vi "Lower_Stop_ms2.vi"(8 "error in (no error)":errorcluster, 10 "I-O in":refnum<class "I-O.lvclass">, 11 "Motion in":refnum<class "Motion.lvclass">) -> (0 "error out":errorcluster, 2 "I-O out":refnum<class "I-O.lvclass">, 3 "Motion out":refnum<class "Motion.lvclass">)   [LabVIEW 2016]
uses:
  Classes/Controller/Motion/Motion Folder/Motion.lvclass
  Classes/Controller/I-O/I-O Folder/I-O.lvclass
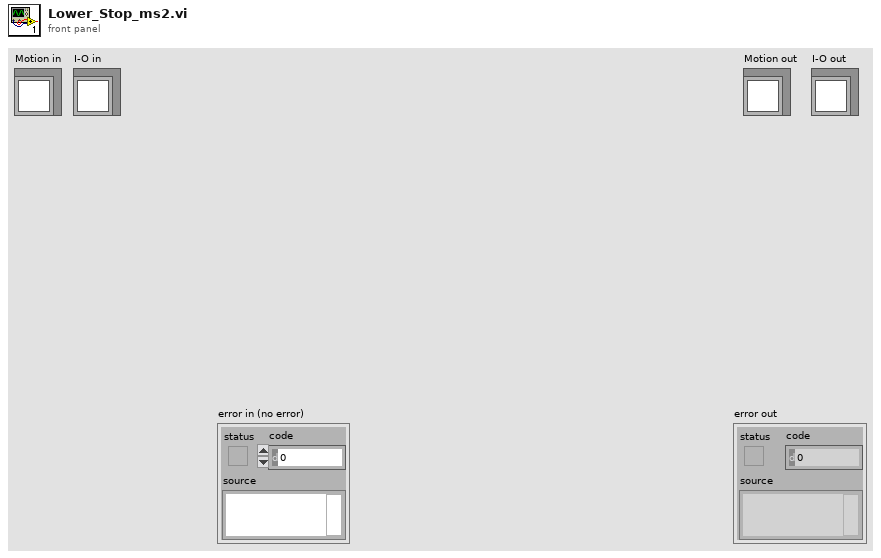
[diagram p1: front panel]
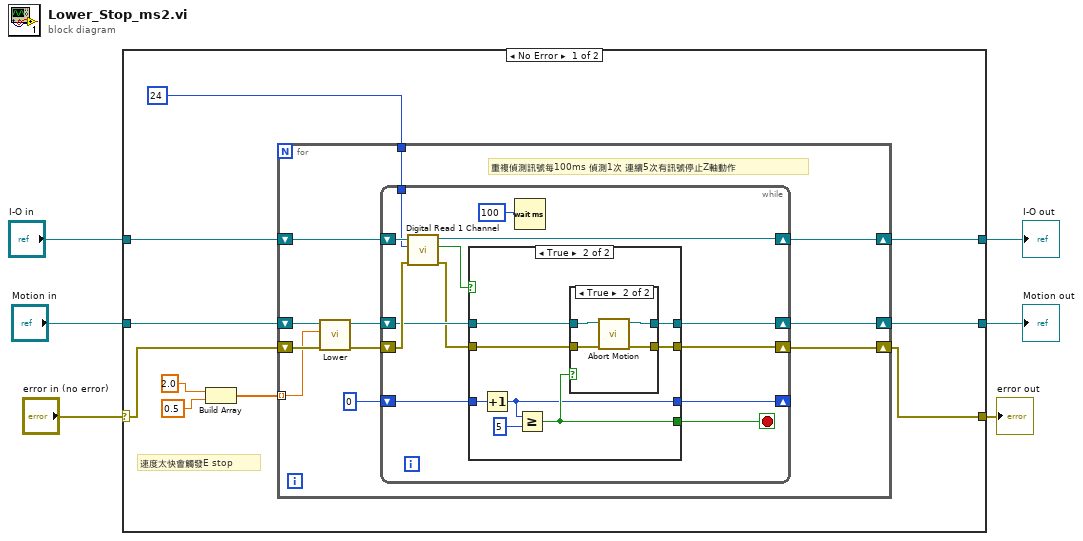
[diagram p0: block diagram]
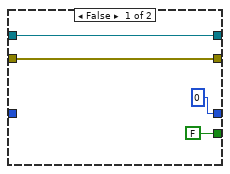
[diagram p2: hidden frame]
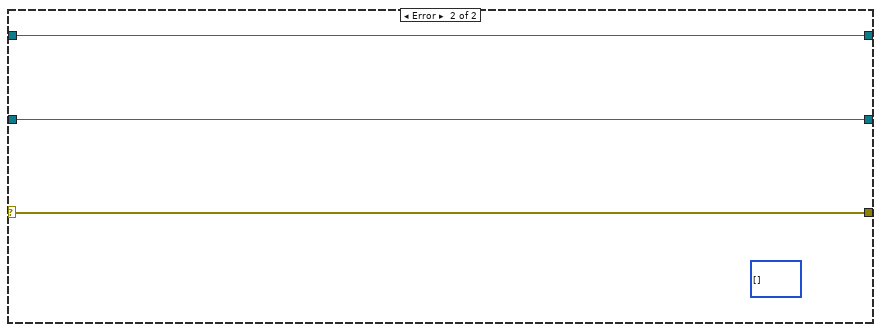
[diagram p4: hidden frame]
diagram:
  n1 = case shown="No Error" "error in (no error)" {
    selector: "error in (no error)" -> [w14 w61]
    tunnel: [w7 w61] -> w5
    tunnel: "Motion in" -> [w16 w60]
    tunnel: "I-O in" -> [w15 w59]
    tunnel: [w9 w60] -> w2
    tunnel: [w8 w59] -> w1
    frame No Error {
      # "速度太快會觸發E stop"
      n2 = Build Array(2.0 ("Speed"), 0.5 ("Speed")) -> (w10:dbl[])
      n3 = for {
        shift-right: [w23] -> w9
        shift-left: w16 -> [w21]
        shift-right: [w27] -> w8
        shift-left: w15 -> [w24]
        shift-right: [w25] -> w7
        shift-left: w14 -> [w18]
        tunnel: 24 ("Read") -> [w26]
        tunnel: w10 -> [w17] mode=indexing
        # "重複偵測訊號每100ms 偵測1次 連續5次有訊號停止Z軸動作"
        n4 = call-dynamic "Lower.vi"("error in (no error)"=w18, "Speed"=w17, "Motion in"=w21) -> ("error out"=w19:errorcluster, "Motion out"=w20:refnum<class "Motion.lvclass">)  [unwired: 7 in]
        n5 = while {
          shift-right: [w39] -> w27
          shift-left: w24 -> [w40]
          tunnel: w26 -> [w37]
          shift-right: [w30] -> w25
          shift-left: w19 -> [w36]
          shift-right: [w32] -> w23
          shift-left: w20 -> [w31]
          shift-right: [w33] -> _
          shift-left: 0 -> [w34]
          stop <- w35 stop-if-true
          n6 = call-dynamic "Digital Read 1 Channel.vi"("error in (no error)"=w36, "Read"=w37, "I-O in"=w40) -> ("error out"=w29:errorcluster, "Value"=w38:bool, "I-O out"=w39:refnum<class "I-O.lvclass">)  [unwired: 6 in]
          n7 = case shown="True" w38 {
            tunnel: [FALSE ("Value") w51] -> w35
            tunnel: w34 -> [_ w50]
            tunnel: [0 w49] -> w33
            tunnel: [w41 w48] -> w32
            tunnel: w31 -> [w41 w47]
            tunnel: [w42 w46] -> w30
            tunnel: w29 -> [w42 w45]
            frame False {
            }
            frame True {
              n8 = Increment(x=w50) -> (x+1=w49:i32)
              n9 = Greater Or Equal?(x=w49, y=5) -> (x >= y?=w51:bool)
              n10 = case shown="True" w51 {
                tunnel: [w53 w58] -> w48
                tunnel: w47 -> [w53 w57]
                tunnel: [w54 w56] -> w46
                tunnel: w45 -> [w54 w55]
                frame False {
                }
                frame True {
                  n11 = call-dynamic "Abort Motion.vi"("error in (no error)"=w55, "Motion in"=w57) -> ("error out"=w56:errorcluster, "Motion out"=w58:refnum<class "Motion.lvclass">)  [unwired: 8 in]
                }
              }
            }
          }
          n12 = Wait (ms)(milliseconds to wait=u32 100) -> ()  [unwired: 1 out]
        }
      }
    }
    frame Error {
      (unwired) u32[][] []
    }
  }
  "error out" <- w5
  "Motion out" <- w2
  "I-O out" <- w1
